vi "Global_Joystick.vi"() -> ()   [LabVIEW 2016]
panel:
  out "Povs":i16[](array[numeric])
  out "Axes":dbl[](array[numeric])
  in  "Buttons":bool[](array[boolean])
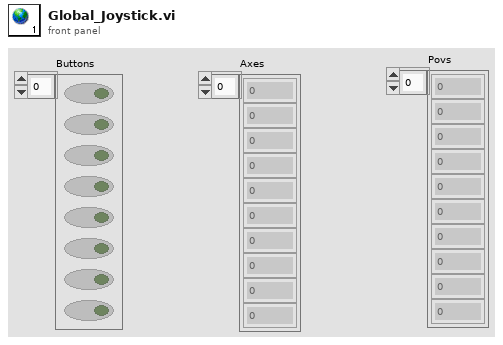
[diagram p1: front panel]
diagram:
